vi "Read from Hardware.vi"(8 "error in":errorcluster, 10 "values in":dbl[](array[numeric]), 11 "logging execution unit in":refnum<class "Logging Execution Unit.lvclass">) -> (0 "error out":errorcluster, 2 "values out":dbl[](array[numeric]), 3 "logging execution unit out":refnum<class "Logging Execution Unit.lvclass">)   [LabVIEW 2020, in "Ballard MIL-STD-1553 Engine.lvlib" / "Implementation.lvlib" / "Logging Execution Unit.lvclass"]
uses:
  Logging Execution Unit.lvclass
  C:/Users/nitest/Desktop/Git 2020/niveristand-aim-milStd1553-custom-device/Source/Custom Device Support/Engine/Implementation/Execution Unit/Execution Unit.lvclass
  Execution Unit/Execution Unit.lvclass/Execution Unit.ctl
  Logging Execution Unit.lvclass/Logging Execution Unit.ctl
  Custom Device/Write Error to System Log.vi/ca55ed61-c1f5-4d13-8aef-490b87d2cf89.vi
  <vilib>/NI VeriStand/Custom Device Tools/Custom Device Utility Library/NI VeriStand - Print Debug Line.vi
  <instrlib>/BTICardLib/BTICardLV.lvlib
  Execution Unit/Execution Unit.lvclass
  Logging/Word Logging/Word Logging.lvlib
  Custom Device/Custom Device.lvlib
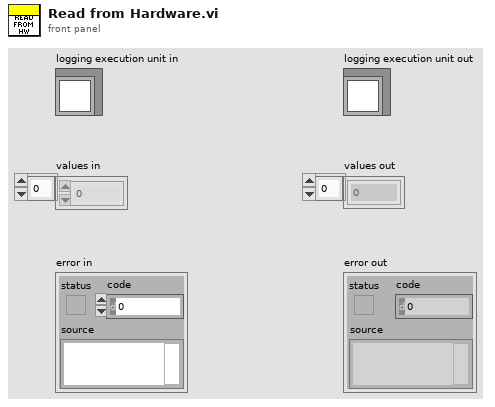
[diagram p1: front panel]
types:
  T1 = typedef "Ballard MIL-STD-1553 Engine.lvlib/Custom Device.lvlib/Hardware Handles.ctl" = cluster{"core handle":u64, "core reader handle":u64, "channel handles":u64[]}
  T2 = typedef "BTICardLV.lvlib/1553 Record.ctl" = cluster{"type":u16, "count":u16, "timestamp":u32, "activity":u16, "error":u16, "cwd1":u16, "cwd2":u16, "swd1":u16, "swd2":u16, "datacount":u16, "data":u16[], "timestamph":u32, "resptime1":u16, "resptime2":u16}
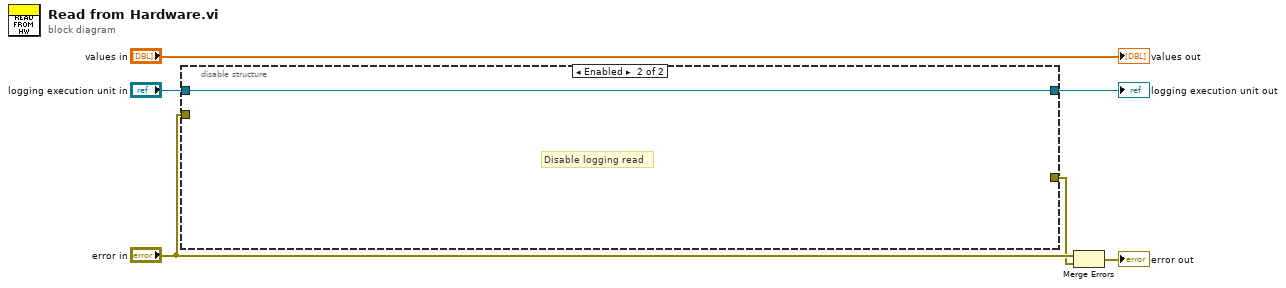
[diagram p0: block diagram]
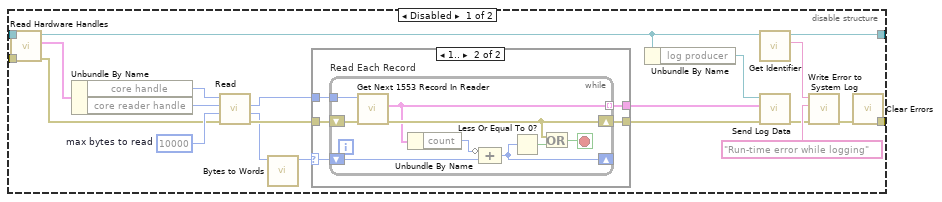
[diagram p2: hidden frame]
diagram:
  n1 = disable-structure shown="Enabled" {
    disable-tunnel: "logging execution unit in" -> [w18 w43]
    disable-tunnel: [w11 w43] -> w4
    disable-tunnel: "error in" -> [w8 _]
    disable-tunnel: [w7 _] -> w2
    frame Disabled {
      w27 = 10000  # max bytes to read
      n2 = call "Read Hardware Handles.vi"("error in"=w8, "Execution Unit in"=w18) -> ("error out"=w26:errorcluster, "hardware handles"=w25:T1, "Execution Unit out"=w12:refnum<class "Logging Execution Unit.lvclass">)  [unwired: 7 in]
      n3 = Unbundle By Name(w25) -> ("core handle"=w22:u64, "core reader handle"=w21:u64)
      n4 = call <instrlib>:"Read.vi"("error in (no error)"=w26, "max bytes to read"=w27, "core reader handle in"=w21, "core handle in"=w22) -> ("error out"=w24:errorcluster, "bytes read"=w19:i32, "core reader handle out"=w23:u64)  [unwired: 4 in, 1 out]
      n5 = call "Bytes to Words.vi"("bytes"=w19) -> ("U16 words"=w20:u16)  [unwired: 10 in]
      n6 = case shown="1.." w20 {
        selector: w20 -> [_ w29]
        tunnel: w24 -> [w28 w33]
        tunnel: [w28 w32] -> w15
        tunnel: w23 -> [_ w31]
        tunnel: [_ w30] -> w17
        frame Default {
        }
        frame 1.. {
          n7 = while "Read Each Record" {
            tunnel: w31 -> [w42]
            tunnel: [w39] -> w30 mode=indexing
            shift-right: [w40] -> w32
            shift-left: w33 -> [w41]
            shift-right: [w37] -> _
            shift-left: w29 -> [w38]
            stop <- w35 stop-if-true
            n8 = call <instrlib>:"Get Next 1553 Record In Reader.vi"("error in (no error)"=w41, "core reader handle in"=w42) -> ("error out"=w40:errorcluster, "record out"=w39:T2)  [unwired: 7 in, 1 out]
            n9 = Unbundle By Name(w39) -> ("count"=w34:u16)
            n10 = Compound Arithmetic op=ADD(invert w34, w38) -> (w37:u16)
            n11 = Less Or Equal To 0?(x=w37) -> (x <= 0?=w36:bool)
            n12 = Or(x=w40, y=w36) -> (x .or. y?=w35:bool)
          }
        }
      }
      n13 = Unbundle By Name(w12) -> ("log producer"=w16:refnum<class "Log Producer.lvclass">)
      n14 = call-dynamic "Get Identifier.vi"("Execution Unit Implementation in"=w12) -> ("Identifier"=w9:string, "Execution Unit Implementation out"=w11:refnum<class "Logging Execution Unit.lvclass">)  [unwired: 8 in, 1 out]
      n15 = call "Send Log Data.vi"("error in"=w15, "Data"=w17, "Producer in"=w16) -> ("error out"=w10:errorcluster)  [unwired: 7 in, 1 out]
      n16 = call "Write Error to System Log.vi"("error in"=w10, "message"="Run-time error while logging", "identifier"=w9) -> ("error out"=w14:errorcluster)  [unwired: 8 in]
      n17 = call <vilib>:"Clear Errors.vi"("error in (no error)"=w14) -> ("error out"=w7:errorcluster)  [unwired: 5 in, 1 out]
    }
    frame Enabled {
      # "Disable logging read"
    }
  }
  "logging execution unit out" <- w4
  n18 = Merge Errors("error in", w2) -> (→"error out":errorcluster)
  "values out" <- "values in"
